vi "NIIE_Dropper.vi"(8 "Error":errorcluster, 10 "Point":T1, 11 "Data":T2={"Class"={"Ants"=refnum, "Layer"=refnum, "Templates"=refnum, "Icon"=refnum, "Glyph"=refnum, "Settings"=refnum, "Tools"=refnum}, "Ref"={"Add Layer"=refnum, "Remove Layer"=refnum, "Line Text"=[], "Body Text Spec"=refnum, "DNL_Font"=refnum, "glyph path str"=refnum, "templates path str"=refnum, "Arrow Up"=refnum, "Arrow Down"=refnum, "IE VI Ref"=refnum, "Glyphs tree"=refnum, "Templates tree"=refnum, "Layer Icon Text"=refnum, "Layer Template"=refnum, "Clipboard"=refnum, "BW icon in"=refnum, "Color icon in"=refnum, "Layer Clust"=refnum, "Body Text"=refnum, "DNL_Framework Templates"=refnum, "Search Templates"=refnum, "TextMarker"=refnum, "Tab Control"=refnum, "Search Glyphs"=refnum, "Line Color"=refnum, "DNL_Glyphs []"=refnum, "Fill Color"=refnum, "Tools"=refnum, "Glyphs tree"=refnum, "Icon"=refnum, "Preview"=refnum, "Ants"=refnum, "Terminals"=refnum, "menu reference"=refnum, "LayerNames"=[], "GlyphLoadAnimation"=refnum, "TemplateLoadAnimation"=refnum, "refreshGlyphs"=refnum, "refreshTemplates"=refnum}, "Support"={"AntsRect"={"left"=0, "top"=0, "right"=0, "bottom"=0}, "Mouse Move Coords"={"Horizontal"=0, "Vertical"=0}, "Mouse Down Coords"={"Horizontal"=0, "Vertical"=0}, "Temp Coord"={"Horizontal"=0, "Vertical"=0}, "Action"=enum."Default", "Edge Color"=4914962, "Fill Color"=16860, "Mouse Down?"=FALSE, "Draft Mode?"=FALSE, "Temp Icon"=bytes[3102], "CTRL Pressed"=FALSE, "Move Selection?"=FALSE, "AntsRect Orig"={"left"=0, "top"=0, "right"=0, "bottom"=0}, "Text"="", "TM Set?"=FALSE, "Mouse inside icon?"=FALSE, "Tool (old value)"=0, "Pencil Move Color"=0, "Swap Colors?"=FALSE, "Shift pressed?"=FALSE}}) -> (0 "Error Out":errorcluster, 2 "Color Out":u32, 3 "Data Out":T2={"Class"={"Ants"=refnum, "Layer"=refnum, "Templates"=refnum, "Icon"=refnum, "Glyph"=refnum, "Settings"=refnum, "Tools"=refnum}, "Ref"={"Add Layer"=refnum, "Remove Layer"=refnum, "Line Text"=[], "Body Text Spec"=refnum, "DNL_Font"=refnum, "glyph path str"=refnum, "templates path str"=refnum, "Arrow Up"=refnum, "Arrow Down"=refnum, "IE VI Ref"=refnum, "Glyphs tree"=refnum, "Templates tree"=refnum, "Layer Icon Text"=refnum, "Layer Template"=refnum, "Clipboard"=refnum, "BW icon in"=refnum, "Color icon in"=refnum, "Layer Clust"=refnum, "Body Text"=refnum, "DNL_Framework Templates"=refnum, "Search Templates"=refnum, "TextMarker"=refnum, "Tab Control"=refnum, "Search Glyphs"=refnum, "Line Color"=refnum, "DNL_Glyphs []"=refnum, "Fill Color"=refnum, "Tools"=refnum, "Glyphs tree"=refnum, "Icon"=refnum, "Preview"=refnum, "Ants"=refnum, "Terminals"=refnum, "menu reference"=refnum, "LayerNames"=[], "GlyphLoadAnimation"=refnum, "TemplateLoadAnimation"=refnum, "refreshGlyphs"=refnum, "refreshTemplates"=refnum}, "Support"={"AntsRect"={"left"=0, "top"=0, "right"=0, "bottom"=0}, "Mouse Move Coords"={"Horizontal"=0, "Vertical"=0}, "Mouse Down Coords"={"Horizontal"=0, "Vertical"=0}, "Temp Coord"={"Horizontal"=0, "Vertical"=0}, "Action"=enum."Default", "Edge Color"=4914962, "Fill Color"=16860, "Mouse Down?"=FALSE, "Draft Mode?"=FALSE, "Temp Icon"=bytes[3102], "CTRL Pressed"=FALSE, "Move Selection?"=FALSE, "AntsRect Orig"={"left"=0, "top"=0, "right"=0, "bottom"=0}, "Text"="", "TM Set?"=FALSE, "Mouse inside icon?"=FALSE, "Tool (old value)"=0, "Pencil Move Color"=0, "Swap Colors?"=FALSE, "Shift pressed?"=FALSE}})   [LabVIEW 2021]
uses:
  Controls/IE Data.ctl
  Class/Ants/Ants.lvclass
  Class/FakedArray/FakedArray.lvclass
  vi.lib/LabVIEW Icon API/lv_icon/Classes/Icon/Icon.lvclass
  Class/Icon Library/Glyph.lvclass
  Class/Settings/Settings.lvclass
  Class/Tools/Tools Paint.lvclass
  Controls/IE Classes.ctl
  Controls/References Cluster.ctl
  Controls/SupportClass.ctl
  <vilib>/Utility/miscctls.llb/LVPoint32TypeDef.ctl
  Controls/ENUM_SupportClass_Action.ctl
  vi.lib/LabVIEW Icon API/lv_icon/Controls/IEColor.ctl
  vi.lib/LabVIEW Icon API/lv_icon/Classes/Icon Framework/Icon Framework.lvclass
  C:/Users/Mark.Balla/Projects/MB Tools/ICON Editor LV/labview-icon-editor-main LV2021 2024-10-24/vi.lib/LabVIEW Icon API/lv_icon/Classes/Layer/Layer.lvclass
  vi.lib/LabVIEW Icon API/lv_icon/Classes/Layer/Layer.lvclass
  vi.lib/LabVIEW Icon API/lv_icon/lv_icon.lvlib
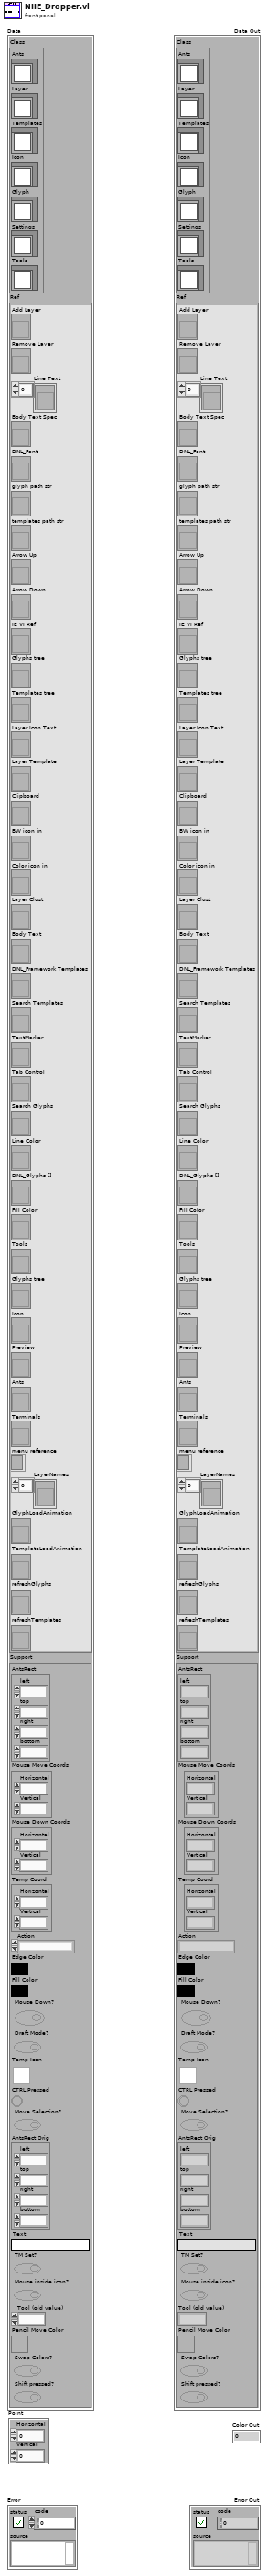
[diagram p1: front panel]
types:
  T1 = typedef "LVPoint32TypeDef.ctl" = cluster{"Horizontal":i32, "Vertical":i32}
  T2 = typedef "IE Data.ctl" = cluster{"Class":T3, "Ref":T4, "Support":T5}
  T3 = typedef "IE Classes.ctl" = cluster{"Ants":refnum<class "Ants.lvclass">, "Layer":refnum<class "FakedArray.lvclass">, "Templates":refnum<class "FakedArray.lvclass">, "Icon":refnum<class "Icon.lvclass">, "Glyph":refnum<class "Glyph.lvclass">, "Settings":refnum<class "Settings.lvclass">, "Tools":refnum<class "Tools Paint.lvclass">}
  T4 = typedef "References Cluster.ctl" = cluster{"Add Layer":refnum<vi>, "Remove Layer":refnum<vi>, "Line Text":refnum<vi>[], "Body Text Spec":refnum<vi>, "DNL_Font":refnum<vi>, "glyph path str":refnum<vi>, "templates path str":refnum<vi>, "Arrow Up":refnum<vi>, "Arrow Down":refnum<vi>, "IE VI Ref":refnum<vi>, "Glyphs tree":refnum<vi>, "Templates tree":refnum<vi>, "Layer Icon Text":refnum<vi>, "Layer Template":refnum<vi>, "Clipboard":refnum<vi>, "BW icon in":refnum<vi>, "Color icon in":refnum<vi>, "Layer Clust":refnum<vi>, "Body Text":refnum<vi>, "DNL_Framework Templates":refnum<vi>, "Search Templates":refnum<vi>, "TextMarker":refnum<vi>, "Tab Control":refnum<vi>, "Search Glyphs":refnum<vi>, "Line Color":refnum<vi>, "DNL_Glyphs []":refnum<vi>, "Fill Color":refnum<vi>, "Tools":refnum<vi>, "Glyphs tree":refnum<vi>, "Icon":refnum<vi>, "Preview":refnum<vi>, "Ants":refnum<vi>, "Terminals":refnum<vi>, "menu reference":refnum<k9>, "LayerNames":refnum<vi>[], "GlyphLoadAnimation":refnum<vi>, "TemplateLoadAnimation":refnum<vi>, "refreshGlyphs":refnum<vi>, "refreshTemplates":refnum<vi>}
  T5 = typedef "SupportClass.ctl" = cluster{"AntsRect":cluster{"left":i16, "top":i16, "right":i16, "bottom":i16}, "Mouse Move Coords":T1, "Mouse Down Coords":T1, "Temp Coord":T1, "Action":T6, "Edge Color":T7, "Fill Color":T7, "Mouse Down?":bool, "Draft Mode?":bool, "Temp Icon":picture, "CTRL Pressed":bool, "Move Selection?":bool, "AntsRect Orig":cluster{"left":i16, "top":i16, "right":i16, "bottom":i16}, "Text":string, "TM Set?":bool, "Mouse inside icon?":bool, "Tool (old value)":u32, "Pencil Move Color":u32, "Swap Colors?":bool, "Shift pressed?":bool}
  T6 = typedef "ENUM_SupportClass_Action.ctl" = enum16{"Default", "Move Selection", "Glyph Library", "Tool"}
  T7 = typedef "IEColor.ctl" = u32
  T8 = typedef "Cluster_Layer Data.ctl" = cluster{"LayerIcon":picture, "LayerName":string, "Opacity":u8, "Visibility?":bool}
  T9 = typedef "LVPositionTypeDef.ctl" = cluster{"Left":i32, "Top":i32}
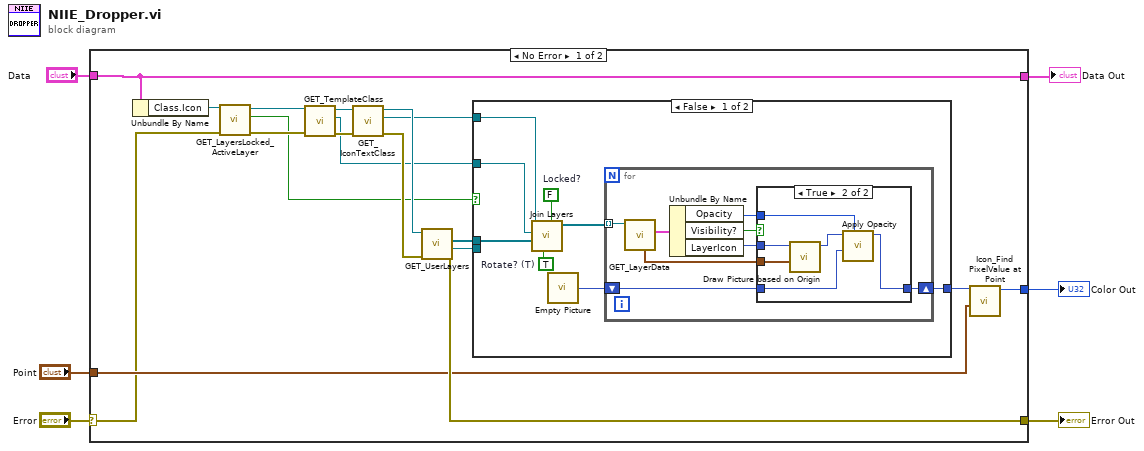
[diagram p0: block diagram]
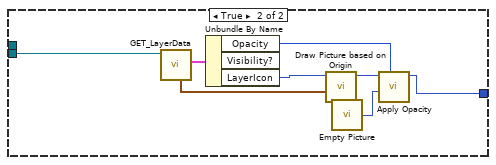
[diagram p3: hidden frame]
diagram:
  n1 = case shown="No Error" "Error" {
    selector: "Error" -> [w8 w57]
    tunnel: [w24 w57] -> w5
    tunnel: "Point" -> [w22 _]
    tunnel: [w21 _] -> w4
    tunnel: "Data" -> [w7 w56]
    tunnel: [w7 w56] -> w2
    frame No Error {
      n2 = Unbundle By Name(w7) -> ("Class.Icon"=w9:refnum<class "Icon.lvclass">)
      n3 = call-dynamic "GET_LayersLocked_ActiveLayer.vi"("error in (no error)"=w8, "Icon.lvclass in"=w9) -> ("error out"=w15:errorcluster, "Layers Locked?"=w11:bool, "Icon.lvclass out"=w16:refnum<class "Icon.lvclass">)  [unwired: 7 out]
      n4 = call-dynamic "GET_TemplateClass.vi"("error in (no error)"=w15, "Icon.lvclass in"=w16) -> ("error out"=w19:errorcluster, "Icon Framework.lvclass"=w13:refnum<class "Icon Framework.lvclass">, "Icon.lvclass out"=w20:refnum<class "Icon.lvclass">)  [unwired: 7 out]
      n5 = call-dynamic "GET_IconTextClass.vi"("error in (no error)"=w19, "Icon.lvclass in"=w20) -> ("error out"=w17:errorcluster, "Icon Framework.lvclass"=w14:refnum<class "Icon Framework.lvclass">, "Icon.lvclass out"=w18:refnum<class "Icon.lvclass">)  [unwired: 7 out]
      n6 = call-dynamic "GET_UserLayers.vi"("error in (no error)"=w17, "Icon.lvclass in"=w18) -> ("error out"=w24:errorcluster, "Active Layer"=w10:refnum<class "Layer.lvclass">, "All Layers"=w12:refnum<class "Layer.lvclass">[])  [unwired: 7 out]
      n7 = case shown="False" w11 {
        tunnel: [w32 w55] -> w23
        tunnel: w14 -> [w29 _]
        tunnel: w13 -> [w28 _]
        tunnel: w12 -> [w27 _]
        tunnel: w10 -> [_ w48]
        frame False {
          w25 = TRUE  # Rotate? (T)
          w26 = FALSE  # Locked?
          n8 = call "Join Layers.vi"("Locked?"=w26, "Rotate? (T)"=w25, "User Layers"=w27, "Template"=w28, "Icon Text"=w29) -> ("Layer Out"=w30:refnum<class "Layer.lvclass">[])  [unwired: 1 in, 5 out]
          n9 = call "Empty Picture"() -> ("empty picture"=w31:picture)
          n10 = for {
            shift-right: [w35] -> w32
            shift-left: w31 -> [w36]
            tunnel: w30 -> [w33] mode=indexing
            n11 = call-dynamic "GET_LayerData.vi"("Layer.lvclass in"=w33) -> ("Data"=w39:T8, "Origin"=w40:T9)  [unwired: 1 in, 8 out]
            n12 = Unbundle By Name(w39) -> ("Opacity"=w37:u8, "Visibility?"=w38:bool, "LayerIcon"=w34:picture)
            n13 = case shown="True" w38 {
              tunnel: w40 -> [_ w47]
              tunnel: w37 -> [_ w46]
              tunnel: w36 -> [w41 w44]
              tunnel: [w41 w43] -> w35
              tunnel: w34 -> [_ w42]
              frame False {
              }
              frame True {
                n14 = call "Draw Picture based on Origin.vi"("Origin"=w47, "LayerIcon in"=w42) -> ("LayerIcon out"=w45:picture)  [unwired: 1 in, 8 out]
                n15 = call "Apply Opacity.vi"("% (100)"=w46, "Bottom"=w44, "Top"=w45) -> ("new picture"=w43:picture)  [unwired: 8 out]
              }
            }
          }
        }
        frame True {
          n16 = call-dynamic "GET_LayerData.vi"("Layer.lvclass in"=w48) -> ("Data"=w52:T8, "Origin"=w53:T9)  [unwired: 1 in, 8 out]
          n17 = Unbundle By Name(w52) -> ("Opacity"=w51:u8, "LayerIcon"=w50:picture)  [unwired: 1 out]
          n18 = call "Draw Picture based on Origin.vi"("Origin"=w53, "LayerIcon in"=w50) -> ("LayerIcon out"=w49:picture)  [unwired: 1 in, 8 out]
          n19 = call "Empty Picture"() -> ("empty picture"=w54:picture)
          n20 = call "Apply Opacity.vi"("% (100)"=w51, "Bottom"=w54, "Top"=w49) -> ("new picture"=w55:picture)  [unwired: 8 out]
        }
      }
      n21 = call "Icon_Find PixelValue at Point.vi"("Point"=w22, "Picture"=w23) -> ("Color Box Out"=w21:u32)  [unwired: 9 out]
    }
    frame Error {
    }
  }
  "Error Out" <- w5
  "Color Out" <- w4
  "Data Out" <- w2
